vi "Update CVT.vi"(8 "error in (no error)":errorcluster, 11 "Measurement in":refnum<class "Measurement.lvclass">) -> (0 "error out":errorcluster, 3 "Measurement out":refnum<class "Measurement.lvclass">)   [LabVIEW 2026, in "Measurement Actor.lvlib" / "Measurement.lvclass"]
uses:
  Measurement.lvclass
  Measurement.lvclass/Measurement.ctl
  recovery/packages/ni_lib_cvt-3.3.0.13-26D4309B9E/File Group 0/vi.lib/NI/Current Value Table/DataTypes/Array of Double_Write.vi
  recovery/packages/ni_lib_cvt-3.3.0.13-26D4309B9E/File Group 0/vi.lib/NI/Current Value Table/Type to Enum.vi
  recovery/packages/ni_lib_cvt-3.3.0.13-26D4309B9E/File Group 0/vi.lib/NI/Current Value Table/DataTypes/Array of Double_Type To Enum.vi
  recovery/packages/ni_lib_cvt-3.3.0.13-26D4309B9E/File Group 0/vi.lib/NI/Current Value Table/FGVs/CVT Globals.vi
  recovery/packages/ni_lib_cvt-3.3.0.13-26D4309B9E/File Group 0/vi.lib/NI/Current Value Table/FGVs/Tag Memory.vi
  recovery/packages/ni_lib_cvt-3.3.0.13-26D4309B9E/File Group 0/vi.lib/NI/Current Value Table/Memory Block.vi
  recovery/packages/ni_lib_cvt-3.3.0.13-26D4309B9E/File Group 0/vi.lib/NI/Current Value Table/DataTypes/Array of Double_Memory Block.vi
  Hardware/Hardware.lvclass
  recovery/packages/ni_lib_cvt-3.3.0.13-26D4309B9E/File Group 0/vi.lib/NI/Current Value Table/Current Value Table.lvlib
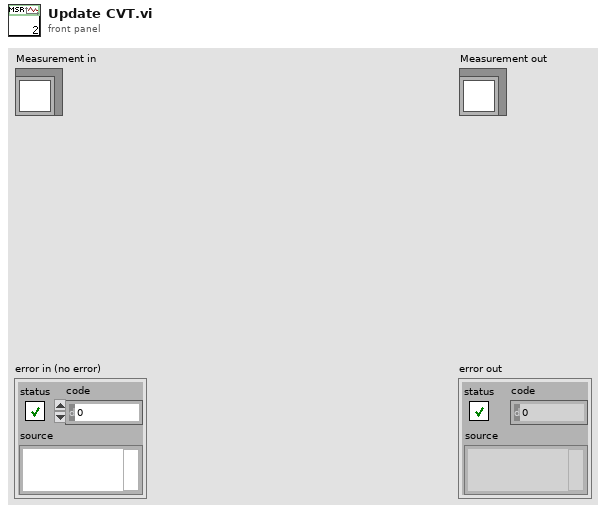
[diagram p1: front panel]
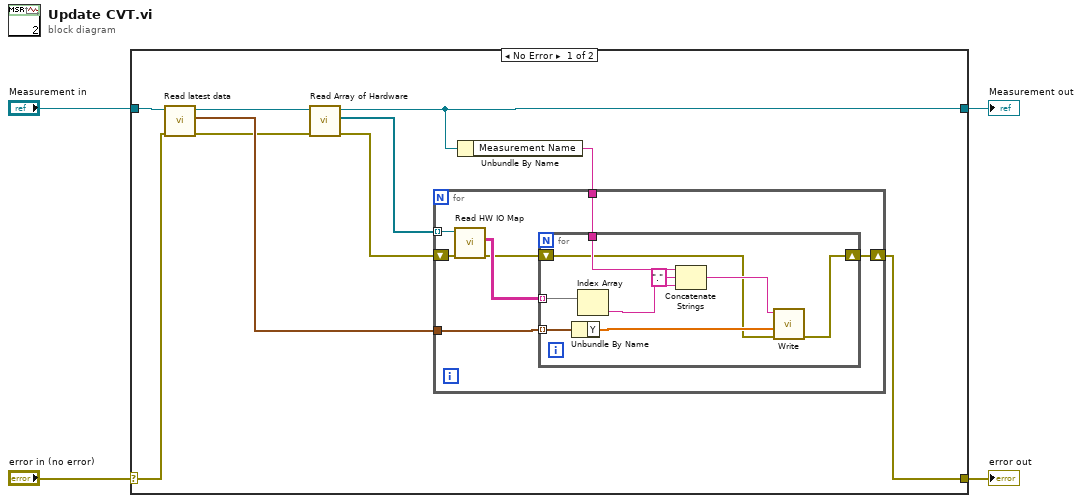
[diagram p0: block diagram]
diagram:
  n1 = case shown="No Error" "error in (no error)" {
    selector: "error in (no error)" -> [w6 w32]
    tunnel: [w5 w32] -> w3
    tunnel: [w10 w31] -> w1
    tunnel: "Measurement in" -> [w12 w31]
    frame No Error {
      n2 = call "Read latest data.vi"("error in (no error)"=w6, "Measurement in"=w12) -> ("error out"=w8:errorcluster, "latest data"=w11:waveform(dbl)[], "Measurement out"=w14:refnum<class "Measurement.lvclass">)  [unwired: 7 in]
      n3 = call "Read Array of Hardware.vi"("error in (no error)"=w8, "Measurement in"=w14) -> ("error out"=w7:errorcluster, "Array of Hardware"=w13:refnum<class "Hardware.lvclass">[], "Measurement out"=w10:refnum<class "Measurement.lvclass">)  [unwired: 7 in]
      n4 = Unbundle By Name(w10) -> ("Measurement Name"=w9:string)
      n5 = for {
        tunnel: w13 -> [w21] mode=indexing
        tunnel: w11 -> [w19]
        tunnel: w9 -> [w18]
        shift-right: [w15] -> w5
        shift-left: w7 -> [w17]
        n6 = call "Read HW IO Map.vi"("error in (no error)"=w17, "Hardware in"=w21) -> ("error out"=w16:errorcluster, "Channel Mapping (Device -> Channel)"=w20:string[][])  [unwired: 7 in, 1 out]
        n7 = for {
          tunnel: w20 -> [w30] mode=indexing
          tunnel: w19 -> [w29] mode=indexing
          tunnel: w18 -> [w27]
          shift-right: [w22] -> w15
          shift-left: w16 -> [w23]
          n8 = Unbundle By Name(w29) -> ("Y"=w28:dbl[])
          n9 = Index Array(array=w30) -> (element=w26:string)  [unwired: 1 in]
          n10 = Concatenate Strings(w27, "." ("string"), w26) -> (w25:string)
          n11 = call-poly "Write.vi"("error in (no error)"=w23, "Value"=w28, "Tag Name"=w25) -> ("error out"=w22:errorcluster)  [unwired: 8 in]
        }
      }
    }
    frame Error {
    }
  }
  "error out" <- w3
  "Measurement out" <- w1
